vi "Disabled.vi"(7 "Robot Mode":T2, 10 "Match Info":T1={"Autonomous Elapsed Seconds"=0.0, "TeleOp Elapsed Seconds"=0.0, "Disabled Elapsed Seconds"=0.0, "Visited Autonomous"=FALSE, "Visited TeleOp"=FALSE, "Visited Disabled"=FALSE, "Autonomous Settings"={"Autonomous Style"=enum."Independent", "VI Refnum"=refnum}}, 11 "Call Context":T3) -> ()   [LabVIEW 2017]
doc: "This VI is called each time a disabled packet is received from the DS. It is often used to prepare for the next robot mode, to calibrate sensors, etc."
uses:
  <vilib>/Rock Robotics/WPI/DriverStation/WPI_DriverStationDerivedRobotMode.ctl
  <vilib>/Rock Robotics/WPI/DriverStation/WPI_DriverStationRobotMode2.ctl
  <vilib>/Rock Robotics/WPI/DriverStation/WPI_DriverStationMatch Info.ctl
  Lift States.ctl
  Robot Global Data.vi
  <vilib>/Rock Robotics/Network Tables/NT Write String Array.vi
  <vilib>/Rock Robotics/Network Tables/NT Read String.vi
  <vilib>/Rock Robotics/Network Tables/NT Read Number.vi
panel:
  in  "Last File Update Time":u32
  out "filenames":string[](array[string])
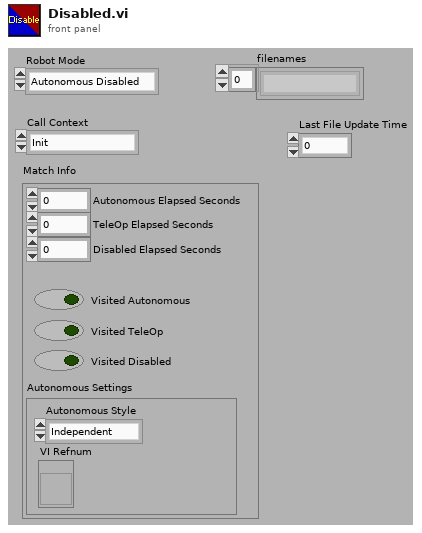
[diagram p1: front panel]
types:
  T1 = typedef "WPI_DriverStationMatch Info.ctl" = cluster{"Autonomous Elapsed Seconds":dbl, "TeleOp Elapsed Seconds":dbl, "Disabled Elapsed Seconds":dbl, "Visited Autonomous":bool, "Visited TeleOp":bool, "Visited Disabled":bool, "Autonomous Settings":cluster{"Autonomous Style":enum16{"Iterative", "Independent"}, "VI Refnum":refnum<vi>}}
  T2 = typedef "WPI_DriverStationRobotMode2.ctl" = enum16{"Autonomous Disabled", "Autonomous Enabled", "Teleop Disabled", "Teleop Enabled", "Disconnected", "Finish", "Test Disabled", "Test Enabled", "Emergency Stopped"}
  T3 = typedef "WPI_DriverStationDerivedRobotMode.ctl" = enum16{"Init", "Execute", "Stop"}
  T4 = typedef "Lift States.ctl" = enum16{"Manual", "Scale Low", "Scale Middle", "Scale High", "Rock Bottom", "Almost Down"}
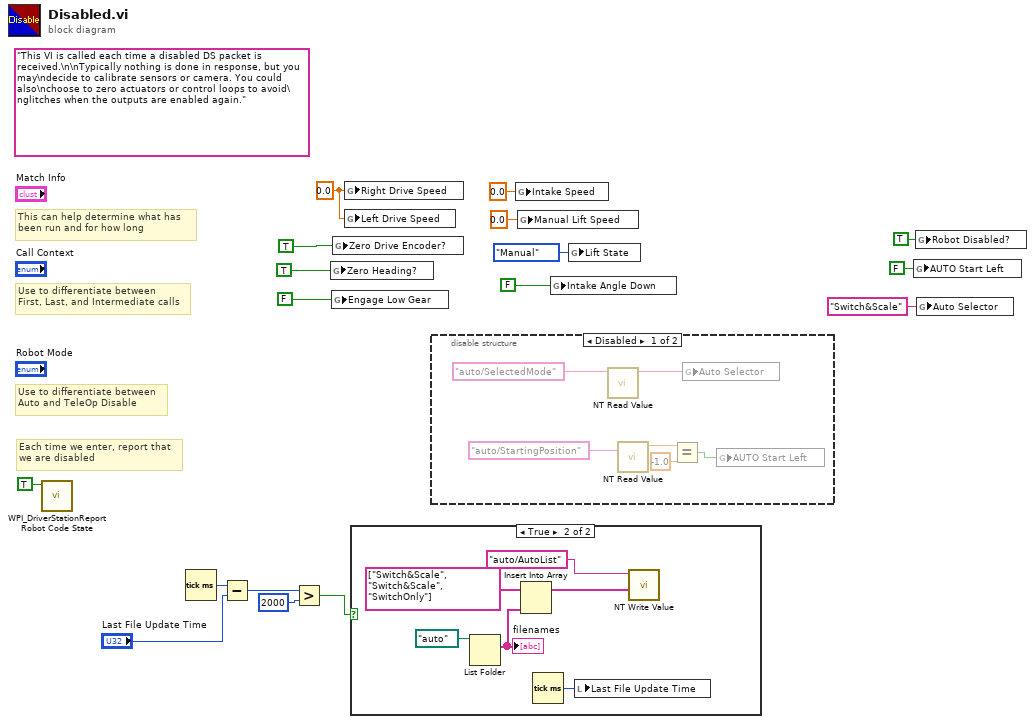
[diagram p0: block diagram]
diagram:
  w15 = 0.0 ("Left Drive Speed")
  (unwired) "This VI is called each time a disabled DS packet is received.\n\nTypically nothing is done in response, but you may\ndecide to calibrate sensors or camera. You could also\nchoose to zero actuators or control loops to avoid\nglitches when the outputs are enabled again."
  # "Each time we enter, report that\nwe are disabled"
  # "Use to differentiate between\nFirst, Last, and Intermediate calls"
  # "This can help determine what has\nbeen run and for how long"
  # "Use to differentiate between\nAuto and TeleOp Disable"
  n1 = call <vilib>:"WPI_DriverStationReport Robot Code State.vi"("Disabled"=TRUE ("Autonomous")) -> ()  [unwired: 10 in, 1 out]
  n2 = Tick Count (ms)() -> (millisecond timer value=w8:u32)
  n3 = Subtract(x=w8, y="Last File Update Time") -> (x-y=w9:u32)
  n4 = Greater?(x=w9, y=u32 2000) -> (0:w5:bool)
  n5 = global write "Robot Global Data.vi" "Zero Heading?"(TRUE ("Zero Heading?")) -> ()
  n6 = global write "Robot Global Data.vi" "Engage Low Gear"(FALSE ("Engage Low Gear")) -> ()
  n7 = global write "Robot Global Data.vi" "Zero Drive Encoder?"(TRUE ("Zero Heading?")) -> ()
  n8 = global write "Robot Global Data.vi" "Right Drive Speed"(w15) -> ()
  n9 = global write "Robot Global Data.vi" "Left Drive Speed"(w15) -> ()
  n10 = case shown="True" w5 {
    frame False {
    }
    frame True {
      n11 = List Folder(path=path "/auto") -> (filenames=w21:string[])  [unwired: 3 in, 3 out]
      "filenames" <- w21
      n12 = Insert Into Array(array=string[] ["Switch&Scale", "Switch&Scale", "SwitchOnly"] ("String Array"), new element=w21) -> (w19:string[])  [unwired: 1 in]
      n13 = Tick Count (ms)() -> (millisecond timer value=w18:u32)
      n14 = local write "Last File Update Time"(w18) -> ()
      n15 = call-poly <vilib>:"NT Write Value.vi"("String Array"=w19, "Name"="auto/AutoList") -> ()  [unwired: 9 in, 1 out]
    }
  }
  n16 = disable-structure shown="Disabled" {
    frame Disabled {
      n17 = call-poly <vilib>:"NT Read Value.vi"("Name"="auto/SelectedMode") -> ("String"=w28:string)  [unwired: 9 in, 1 out]
      n18 = call-poly <vilib>:"NT Read Value.vi"("Name"="auto/StartingPosition") -> ("Numeric"=w26:dbl)  [unwired: 9 in, 1 out]
      n19 = Equal?(x=w26, y=-1.0) -> (x = y?=w24:bool)
      n20 = global write "Robot Global Data.vi" "Auto Selector"(w28) -> ()
      n21 = global write "Robot Global Data.vi" "AUTO Start Left"(w24) -> ()
    }
    frame Enabled {
    }
  }
  n22 = global write "Robot Global Data.vi" "Intake Speed"(0.0 ("Intake Speed")) -> ()
  n23 = global write "Robot Global Data.vi" "Manual Lift Speed"(0.0 ("Intake Speed")) -> ()
  n24 = global write "Robot Global Data.vi" "Intake Angle Down"(FALSE ("Engage Low Gear")) -> ()
  n25 = global write "Robot Global Data.vi" "Lift State"(Lift_States."Manual" ("Lift State")) -> ()
  n26 = global write "Robot Global Data.vi" "AUTO Start Left"(FALSE ("AUTO Start Left")) -> ()
  n27 = global write "Robot Global Data.vi" "Robot Disabled?"(TRUE ("AUTO Start Left")) -> ()
  n28 = global write "Robot Global Data.vi" "Auto Selector"("Switch&Scale" ("Auto Selector")) -> ()
